vi "Leggi coeff motore.vi"(10 "motore":string, 11 "Enum":enum16{"LEGGI COEFF", "INIZIALIZZA"}(ring)) -> (0 "Param motore":T1, 1 "lista MOTORI":string[](array[string]), 2 "coeff":dbl[](array[numeric]))   [LabVIEW 2016]
uses:
  Global percorso impostazioni.vi
  <vilib>/addons/_office/excel.llb/Excel Get Data ([str]).vi
  <vilib>/Utility/NIReport.llb/NI_report.lvclass
  <vilib>/addons/_office/NI_ReportGenerationToolkit.lvlib
  <vilib>/Utility/NIReport.llb/Excel/NI_Excel.lvclass
panel:
  out "data":string[][](array[string])
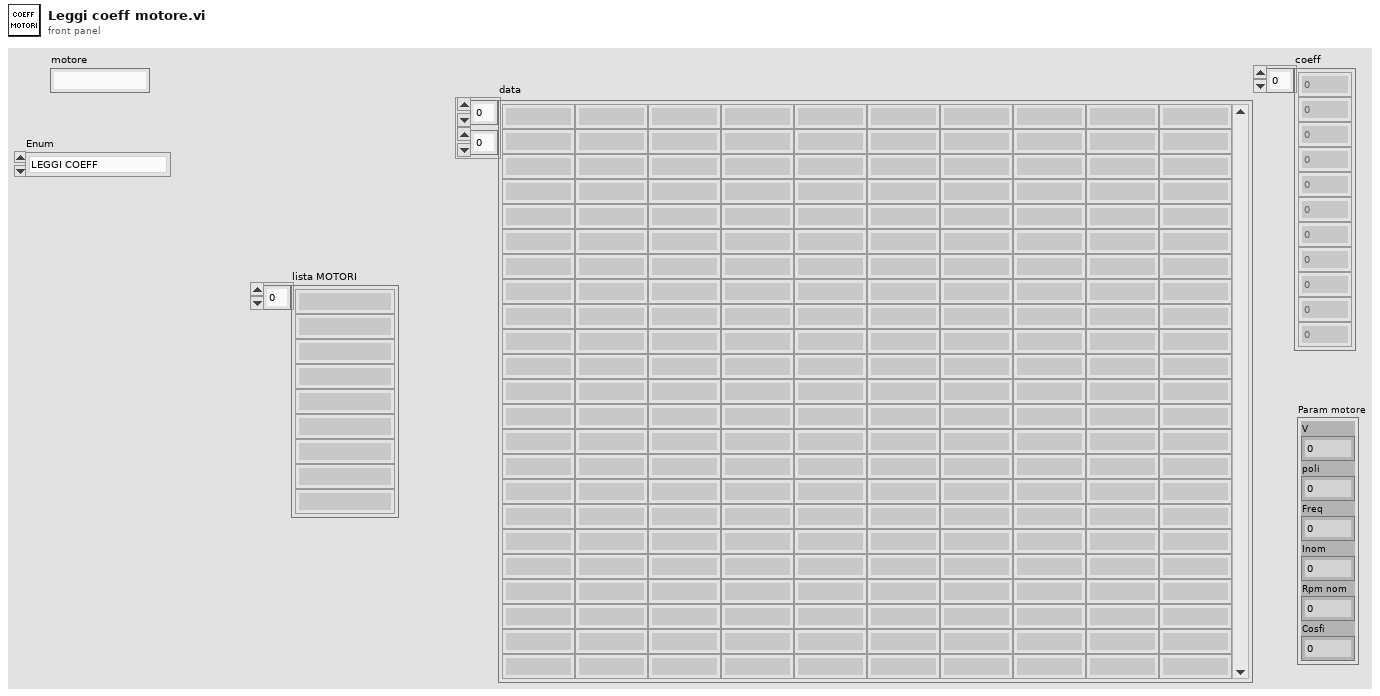
[diagram p1: front panel]
types:
  T1 = cluster{"V":dbl, "poli":dbl, "Freq":dbl, "Inom":dbl, "Rpm nom":dbl, "Cosfi":dbl}
  T2 = enum16{"maximized", "minimized", "normal", "no change"}
  T3 = enum16{"Standard Report", "HTML", "Word", "Excel"}
  T4 = cluster{"[0]":dbl, "[1]":dbl, "[2]":dbl, "[3]":dbl, "[4]":dbl, "[5]":dbl}
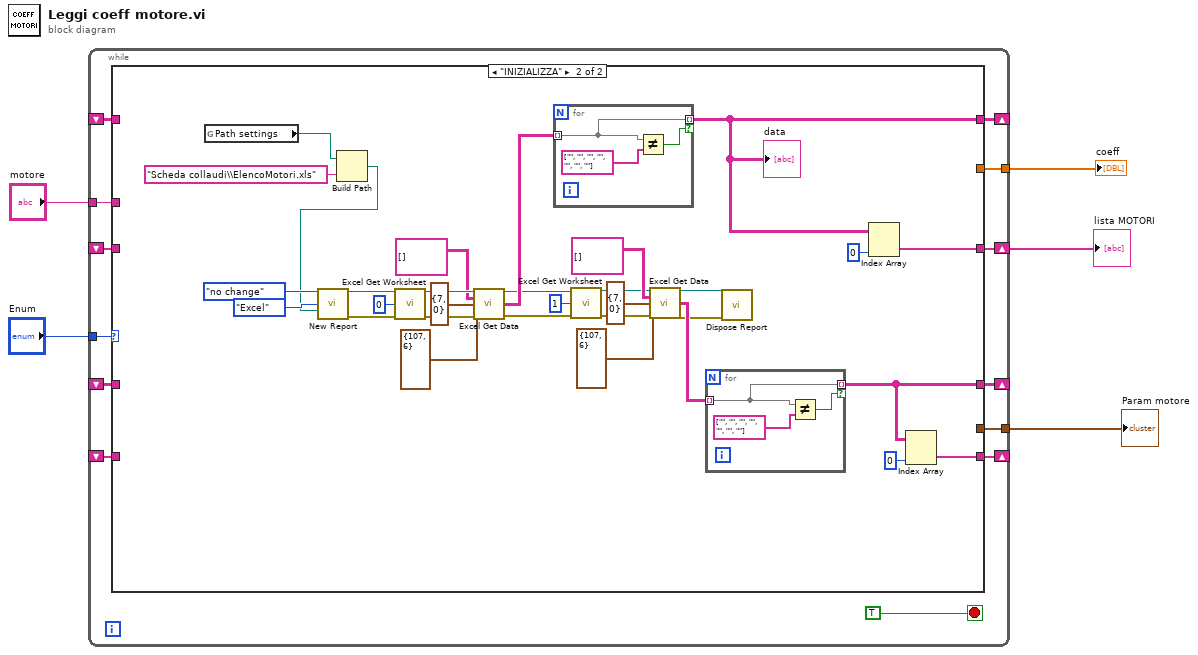
[diagram p0: block diagram]
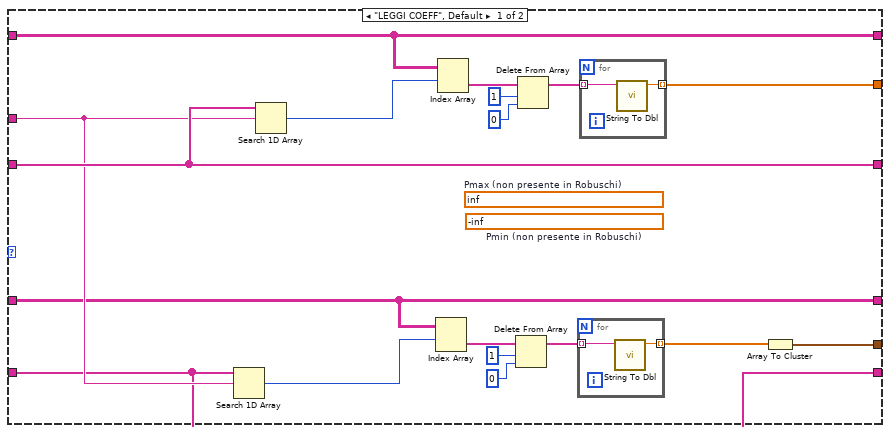
[diagram p2: hidden frame]
diagram:
  n1 = while {
    tunnel: "Enum" -> [w16]
    shift-right: [w15] -> _
    shift-left: _ -> [w13]
    shift-right: [w18] -> w5
    shift-left: _ -> [w14]
    tunnel: [w12] -> w3
    tunnel: "motore" -> [w11]
    shift-right: [w10] -> _
    shift-left: _ -> [w7]
    shift-right: [w9] -> _
    shift-left: _ -> [w8]
    tunnel: [w6] -> w1
    stop <- TRUE stop-if-true
    n2 = case shown="\"INIZIALIZZA\"" w16 {
      tunnel: [w31 w59] -> w18
      tunnel: [w36 w58] -> w15
      tunnel: w14 -> [w31 _]
      tunnel: w13 -> [w36 _]
      tunnel: [w29 _] -> w12
      tunnel: w11 -> [w28 _]
      tunnel: [w23 w44] -> w10
      tunnel: [w21 w43] -> w9
      tunnel: w8 -> [w21 _]
      tunnel: w7 -> [w23 _]
      tunnel: [w19 _] -> w6
      frame "LEGGI COEFF", Default {
        (unwired) -inf  # Pmin (non presente in Robuschi)
        (unwired) inf  # Pmax (non presente in Robuschi)
        n3 = Search 1D Array(1D array=w21, element=w28) -> (index of element=w22:i32)  [unwired: 1 in]
        n4 = Search 1D Array(1D array=w31, element=w28) -> (index of element=w30:i32)  [unwired: 1 in]
        n5 = Index Array(array=w23, index (row)=w22) -> (element=w24:string[])  [unwired: 1 in]
        n6 = Index Array(array=w36, index (row)=w30) -> (element=w35:string[])  [unwired: 1 in]
        n7 = Delete From Array(array=w24, length=1, index=0) -> (array with subset deleted=w27:string[])  [unwired: 1 out]
        n8 = Delete From Array(array=w35, length=1, index=0) -> (array with subset deleted=w32:string[])  [unwired: 1 out]
        n9 = for {
          tunnel: w27 -> [w38] mode=indexing
          tunnel: [w37] -> w20 mode=indexing
          n10 = call "String To Dbl.vi"("String"=w38) -> ("Numeric"=w37:dbl)  [unwired: 10 in]
        }
        n11 = for {
          tunnel: w32 -> [w40] mode=indexing
          tunnel: [w39] -> w29 mode=indexing
          n12 = call "String To Dbl.vi"("String"=w40) -> ("Numeric"=w39:dbl)  [unwired: 10 in]
        }
        n13 = Array To Cluster(array=w20) -> (cluster=w19:T4)
      }
      frame "INIZIALIZZA" {
        n14 = global read "Global percorso impostazioni.vi" "Path settings"() -> (w56:path)
        n15 = Build Path(base path=w56, name or relative path="Scheda collaudi\\ElencoMotori.xls") -> (appended path=w55:path)
        n16 = call <vilib>:"New Report.vi"("window state (normal)"=T2."no change", "report type"=T3."Excel", "template (empty)"=w55) -> ("report out"=w70:refnum<class "NI_report.lvclass">, "error out"=w71:errorcluster)  [unwired: 11 in]
        n17 = call <vilib>:"Excel Get Worksheet.vi"("report in"=w70, "worksheet index (0)"=0, "error in (no error)"=w71) -> ("report out"=w69:refnum<class "NI_report.lvclass">, "error out"=w68:errorcluster)  [unwired: 11 in]
        n18 = call-poly <vilib>:"Excel Get Data.vi"("report in"=w69, "data type"=string[][] [], "start (-1, -1)"=cluster{"start row":i32, "start column":i32} {"start row"=7, "start column"=0} ("start (0, 0)"), "end (-1, -1)"=cluster{"row":i32, "column":i32} {"row"=107, "column"=6}, "error in (no error)"=w68) -> ("report out"=w48:refnum<class "NI_report.lvclass">, "data"=w61:string[][], "error out"=w47:errorcluster)  [unwired: 8 in]
        n19 = for {
          tunnel: w61 -> [w77] mode=indexing
          tunnel: [w77] -> w58 mode=indexing if=w76
          n20 = Not Equal?(x=w77, y=string[] ["", "", "", "", "", "", ""] ("subarray")) -> (x != y?=w76:bool)
        }
        "data" <- w58
        n21 = call <vilib>:"Excel Get Worksheet.vi"("report in"=w48, "worksheet index (0)"=1, "error in (no error)"=w47) -> ("report out"=w49:refnum<class "NI_report.lvclass">, "error out"=w50:errorcluster)  [unwired: 11 in]
        n22 = call-poly <vilib>:"Excel Get Data.vi"("report in"=w49, "data type"=string[][] [], "start (-1, -1)"=cluster{"start row":i32, "start column":i32} {"start row"=7, "start column"=0} ("start (0, 0)"), "end (-1, -1)"=cluster{"row":i32, "column":i32} {"row"=107, "column"=6}, "error in (no error)"=w50) -> ("report out"=w42:refnum<class "NI_report.lvclass">, "data"=w46:string[][], "error out"=w41:errorcluster)  [unwired: 8 in]
        n23 = for {
          tunnel: w46 -> [w74] mode=indexing
          tunnel: [w74] -> w44 mode=indexing if=w73
          n24 = Not Equal?(x=w74, y=string[] ["", "", "", "", "", "", ""] ("subarray")) -> (x != y?=w73:bool)
        }
        n25 = call-dynamic "Dispose Report.vi"("report in"=w42, "error in (no error)"=w41) -> ()  [unwired: 13 in, 1 out]
        n26 = Index Array(array=w58, index (col)=0 ("disabled index (col)")) -> (element=w59:string[])  [unwired: 1 in]
        n27 = Index Array(array=w44, index (col)=0 ("disabled index (col)")) -> (element=w43:string[])  [unwired: 1 in]
      }
    }
  }
  "lista MOTORI" <- w5
  "coeff" <- w3
  "Param motore" <- w1
